vi "getDefault.vi"(7 "String":string, 8 "var number":dbl, 9 "location":dbl, 10 "defaults":string, 11 "value":string) -> (1 "var number 2":dbl, 2 "value 2":string)   [LabVIEW 2012]
panel:
  out "defaults array":string[](array[string])
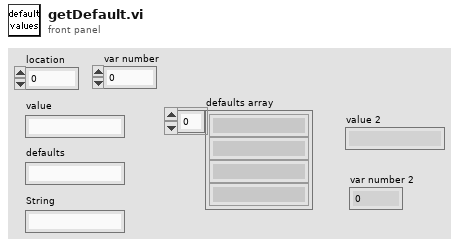
[diagram p1: front panel]
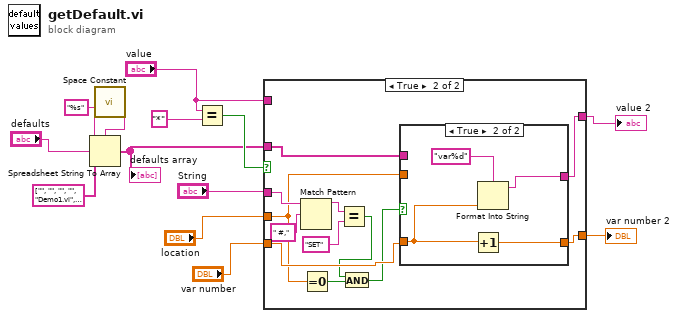
[diagram p0: block diagram]
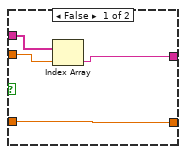
[diagram p3: hidden frame]
diagram:
  n1 = call <vilib>:"Space Constant.vi"() -> ("String"=w5:string)
  n2 = Spreadsheet String To Array(delimiter (Tab)=w5, format string="%s", spreadsheet string="defaults", array type (2D Dbl)=string[] ["", "", "", "", "Demo1.vi", "DigitalWrite.vi", "VS_Wait.vi", ""] ("Array 3")) -> (array=w4:string[])
  "defaults array" <- w4
  n3 = Equal?(x="value", y="*") -> (x = y?=w12:bool)
  n4 = case shown="True" w12 {
    tunnel: "value" -> [w15 _]
    tunnel: "location" -> [_ w19]
    tunnel: [w15 w23] -> w9
    tunnel: w4 -> [_ w24]
    tunnel: "var number" -> [w14 w22]
    tunnel: [w14 w21] -> w2
    tunnel: "String" -> [_ w27]
    frame False {
    }
    frame True {
      n5 = Match Pattern(string=w27, regular expression=" #,") -> (before substring=w25:string)  [unwired: 1 in, 3 out]
      n6 = Equal To 0?(x=w19) -> (x = 0?=w18:bool)
      n7 = Equal?(x=w25, y="SET") -> (x = y?=w17:bool)
      n8 = And(x=w17, y=w18) -> (x .and. y?=w16:bool)
      n9 = case shown="True" w16 {
        tunnel: w24 -> [w31 _]
        tunnel: w19 -> [w30 _]
        tunnel: [w29 w34] -> w23
        tunnel: w22 -> [w28 w33]
        tunnel: [w28 w32] -> w21
        frame False {
          n10 = Index Array(array=w31, index=w30) -> (element=w29:string)
        }
        frame True {
          n11 = Increment(x=w33) -> (x+1=w32:dbl)
          n12 = Format Into String(format string="var%d", w33) -> (resulting string=w34:string)  [unwired: 2 in, 1 out]
        }
      }
    }
  }
  "value 2" <- w9
  "var number 2" <- w2
